vi "LSMcontroller_v66_improvedwfhandling.vi"() -> ()   [LabVIEW 2015] (continued)
                              }
                            }
                            n2122 = property on="Start" class="Bool (strict)"("Val(Sgnl)"=w5239) -> ()  [unwired: 2 in, 2 out]
                            n2123 = property on="Start" class="Bool (strict)"("Visible"=TRUE, "DisabledEnum"=T7."Enabled" ("Disabled")) -> ()  [unwired: 2 in, 2 out]
                            n2124 = property on="Stop" class="Bool (strict)"("Val(Sgnl)"=w5239) -> ()  [unwired: 2 in, 2 out]
                            n2125 = property on="Stop" class="Bool (strict)"("Visible"=FALSE, "DisabledEnum"=T7."Disabled" ("Disabled")) -> ()  [unwired: 2 in, 2 out]
                          }
                        }
                      }
                      frame Enabled {
                      }
                    }
                    n2126 = local write "64bit disabled"(TRUE ("64bit disabled")) -> ()
                  }
                }
              }
            }
          }
          event "avpp", "Angle ref", "xpixels ref", "Vx-min ref", "Vx-max ref", "ypixels ref", "Vy-min ref", "Vy-max ref", "ROI Type", "Sampling rate": Value Change {
            n2127 = event-data() -> ()  [unwired: 1 in, 6 out]
            n2128 = local read "avpp"() -> (w5258:i32)
            n2129 = local read "Angle ref"() -> (w5257:dbl)
            n2130 = local read "ROI Type"() -> (w5256:u16)
            n2131 = local read "xpixels ref"() -> (w5253:i32)
            n2132 = local read "Vx-min ref"() -> (w5252:dbl)
            n2133 = local read "Vx-max ref"() -> (w5251:dbl)
            n2134 = local read "ypixels ref"() -> (w5249:i32)
            n2135 = local read "Vy-min ref"() -> (w5250:dbl)
            n2136 = local read "Vy-max ref"() -> (w5246:dbl)
            n2137 = local read "Sampling rate"() -> (w5241:dbl)
            n2138 = local read "# of frames"() -> (w5245:i32)
            n2139 = local read "maxbufferAI"() -> (w5244:i32)
            n2140 = local read "Override AI buffer"() -> (w5242:bool)
            n2141 = call "2pparameters.vi"("command"="get") -> ("params out"=w5255:T10)  [unwired: 1 in]
            n2142 = Bundle By Name(cluster=w5255, "avpp"=w5258, "Angle Img"=w5257, "Xpixels Img"=w5253, "Vx-min Img"=w5252, "VX-max Img"=w5251, "Ypixels Img"=w5249, "Vy-min Img"=w5250, "Vy-max Img"=w5246, "srate"=w5241, "srate Img"=w5241, "measpoints"=w5245, "maxbufferAI"=w5244, "Drawing Mode"=w5256, "Vz-reset"=0.0, "AIoverride"=w5242) -> (w5247:T10)
            n2143 = call "2pparameters.vi"("Params in"=w5247, "command"="set") -> ()  [unwired: 1 out]
          }
          event "# of frames": Value Change {
            n2144 = event-data() -> ()  [unwired: 1 in, 6 out]
            n2145 = local read "Meastab"() -> (w5259:enum32{"X-Y Image", "Linescan", "Timetrace"})
            n2146 = case shown="\"X-Y Image\", Default" w5259 {
              frame "X-Y Image", Default {
                n2147 = local read "# of frames"() -> (w5260:i32)
                n2148 = call "2pparameters.vi"("command"="get") -> ("params out"=w5264:T10)  [unwired: 1 in]
                n2149 = Bundle By Name(cluster=w5264, "measpoints"=w5260) -> (w5261:T10)
                n2150 = call "2pparameters.vi"("Params in"=w5261, "command"="set") -> ()  [unwired: 1 out]
              }
              frame "Linescan" {
                n2151 = local read "srateAODOtt"() -> (w5274:dbl)
                n2152 = local read "# of frames"() -> (w5270:i32)
                n2153 = local read "refreshtime"() -> (w5276:dbl)
                n2154 = local read "bin"() -> (w5271:dbl)
                n2155 = call "tt_timeandsamples.vi"("bin"=w5271, "refreshtime"=w5276, "srateAODOtt"=w5274, "tot#ofsamples"=w5270) -> ("refreshrate"=w5273:dbl, "refreshbuffer"=w5272:i32, "timetracecycles"=w5269:i32)  [unwired: 5 in]
                n2156 = call "2pparameters.vi"("command"="get") -> ("params out"=w5266:T10)  [unwired: 1 in]
                n2157 = Bundle By Name(cluster=w5266, "measpoints"=w5270, "tt_cycles"=w5269, "refreshbuffer"=w5272, "refreshrate"=w5273) -> (w5268:T10)
                n2158 = Reciprocal(x=w5273) -> (1/x=w5275:dbl)
                n2159 = local write "refreshtime"(w5275) -> ()
                n2160 = call "2pparameters.vi"("Params in"=w5268, "command"="set") -> ()  [unwired: 1 out]
              }
              frame "Timetrace" {
                n2161 = local read "srateAODOtt"() -> (w5286:dbl)
                n2162 = local read "# of frames"() -> (w5282:i32)
                n2163 = local read "refreshtime"() -> (w5288:dbl)
                n2164 = local read "bin"() -> (w5283:dbl)
                n2165 = call "tt_timeandsamples.vi"("bin"=w5283, "refreshtime"=w5288, "srateAODOtt"=w5286, "tot#ofsamples"=w5282) -> ("refreshrate"=w5285:dbl, "refreshbuffer"=w5284:i32, "timetracecycles"=w5281:i32)  [unwired: 5 in]
                n2166 = call "2pparameters.vi"("command"="get") -> ("params out"=w5278:T10)  [unwired: 1 in]
                n2167 = Bundle By Name(cluster=w5278, "measpoints"=w5282, "tt_cycles"=w5281, "refreshbuffer"=w5284, "refreshrate"=w5285) -> (w5280:T10)
                n2168 = Reciprocal(x=w5285) -> (1/x=w5287:dbl)
                n2169 = local write "refreshtime"(w5287) -> ()
                n2170 = call "2pparameters.vi"("Params in"=w5280, "command"="set") -> ()  [unwired: 1 out]
              }
            }
          }
          event "srateAODOtt", "refreshtime", "Vx-ref", "Vy-ref", "Vx-min draw", "Vx-max draw", "Vy-min draw", "Vy-max draw", "bin": Value Change {
            n2171 = event-data() -> ()  [unwired: 1 in, 6 out]
            n2172 = local read "ypixels ref"() -> (w5320:i32)
            n2173 = local read "Vy-min draw"() -> (w5296:dbl)
            n2174 = local read "Vy-max draw"() -> (w5295:dbl)
            n2175 = local read "Vx-min draw"() -> (w5298:dbl)
            n2176 = local read "Vx-max draw"() -> (w5297:dbl)
            n2177 = local read "xpixels ref"() -> (w5294:i32)
            n2178 = local read "ROI Type"() -> (w5293:u16)
            n2179 = local read "Pel"() -> (w5292:dbl)
            n2180 = local read "srateAODOtt"() -> (w5302:dbl)
            n2181 = local read "# of frames"() -> (w5307:i32)
            n2182 = local read "refreshtime"() -> (w5300:dbl)
            n2183 = local read "bin"() -> (w5305:dbl)
            n2184 = local read "Override AI buffer"() -> (w5290:bool)
            n2185 = local read "finite samples"() -> (w5314:bool)
            n2186 = local read "srateAODOtt"() -> (w5289:dbl)
            n2187 = local read "srateAODOtt"() -> (w5308:dbl)
            n2188 = local read "continuous"() -> (w5313:bool)
            n2189 = local read "Angle ref"() -> (w5299:dbl)
            n2190 = local read "wavdet"() -> (w5315:bool)
            n2191 = local read "Vx-ref"() -> (w5310:dbl)
            n2192 = local read "Vy-ref"() -> (w5312:dbl)
            n2193 = local read "avpp"() -> (w5311:i32)
            n2194 = call "tt_timeandsamples.vi"("bin"=w5305, "refreshtime"=w5300, "srateAODOtt"=w5302, "tot#ofsamples"=w5307) -> ("refreshrate"=w5303:dbl, "refreshbuffer"=w5304:i32, "timetracecycles"=w5309:i32)  [unwired: 5 in]
            n2195 = local read "bin"() -> (w5306:dbl)
            n2196 = call "2pparameters.vi"("command"="get") -> ("params out"=w5318:T10)  [unwired: 1 in]
            n2197 = Bundle By Name(cluster=w5318, "Drawing Mode"=w5293, "measpoints"=w5307, "tt_cycles"=w5309, "refreshbuffer"=w5304, "refreshrate"=w5303, "Vx-ref"=w5310, "Vy-ref"=w5312, "srate"=w5289, "finite"=w5314, "cont"=w5313, "wavdet"=w5315, "avpp"=w5311, "srateAODO"=w5308, "bufferAI"=w5304, "bin"=w5306, "Angle Img"=w5299, "Vxminref"=w5298, "Vxmaxref"=w5297, "Vyminref"=w5296, "Vymaxref"=w5295, "Xpixels Img"=w5294, "Ypixels Img"=w5320, "Pel"=w5292, "Vz-reset"=0.0, "AIoverride"=w5290) -> (w5316:T10)
            n2198 = Reciprocal(x=w5303) -> (1/x=w5301:dbl)
            n2199 = local write "refreshtime"(w5301) -> ()
            n2200 = call "2pparameters.vi"("Params in"=w5316, "command"="set") -> ()  [unwired: 1 out]
          }
          event "Init": Value Change {
            # "Disabled for conversion to 64 bit"
            n2201 = event-data() -> ()  [unwired: 1 in, 6 out]
            n2202 = disable-structure shown="Disabled" {
              frame Disabled {
                n2203 = flat-sequence {
                  frame #0 {
                    n2204 = local read "Measurement"() -> (w5322:T4)
                    n2205 = case shown="\"Lifetime (scan)\", \"Lifetime (contour)\"" w5322 {
                      frame "X-Y-t movie", Default {
                      }
                      frame "Lifetime (point)" {
                        n2206 = stacked-sequence {
                          frame #0 {
                            n2207 = call "initialize.vi"("mode"=0) -> ()
                          }
                          frame #1 {
                            n2208 = call "calib.vi"() -> ()  [unwired: 1 in]
                          }
                        }
                      }
                      frame "Lifetime (scan)", "Lifetime (contour)" {
                        n2209 = stacked-sequence {
                          frame #0 {
                            n2210 = call "initialize.vi"("mode"=3) -> ()
                          }
                          frame #1 {
                            n2211 = call "calib.vi"() -> ()  [unwired: 1 in]
                          }
                        }
                      }
                    }
                  }
                  frame #1 {
                    n2212 = property on="Start" class="Bool (strict)"("Visible"=TRUE, "DisabledEnum"=T7."Enabled" ("Disabled")) -> ()  [unwired: 2 in, 2 out]
                    n2213 = property on="Init" class="Bool (strict)"("Visible"=FALSE, "DisabledEnum"=T7."Disabled and Grayed Out" ("Disabled"), "Value"=FALSE ("Init")) -> ()  [unwired: 2 in, 2 out]
                  }
                }
              }
              frame Enabled {
              }
            }
            n2214 = local write "64bit disabled"(TRUE ("64bit disabled")) -> ()
          }
          event "Measurement": Value Change {
            n2215 = event-data() -> ()  [unwired: 1 in, 5 out]
            n2216 = case shown="\"Lifetime (scan)\"" "Measurement" {
              frame "X-Y-t movie" {
                w5337 = T7."Disabled" ("Disabled")
                w5336 = FALSE ("Visible")
                n2217 = call "2pparameters.vi"("command"="get") -> ("params out"=w5347:T10)  [unwired: 1 in]
                n2218 = local write "graphtab"(T5."image" ("graphtab")) -> ()
                n2219 = local write "Save tab"(enum32{"withsave", "withoutsave"}."withsave" ("Save tab")) -> ()
                n2220 = Bundle By Name(cluster=w5347, "type"="X-Y-t movie") -> (w5345:T10)
                n2221 = call "2pparameters.vi"("Params in"=w5345, "command"="set") -> ()  [unwired: 1 out]
                n2222 = property on="refreshtime" class="DigNum (strict)"("Visible"=FALSE, "DisabledEnum"=T7."Disabled and Grayed Out" ("Disabled")) -> ()  [unwired: 2 in, 2 out]
                n2223 = property on="Start" class="Bool (strict)"("Visible"=TRUE, "DisabledEnum"=T7."Enabled" ("Disabled")) -> ()  [unwired: 2 in, 2 out]
                n2224 = property on="Init" class="Bool (strict)"("Visible"=FALSE, "DisabledEnum"=T7."Disabled and Grayed Out" ("Disabled"), "Value"=FALSE ("Init")) -> ()  [unwired: 2 in, 2 out]
                n2225 = property on="ttt" class="Enum (strict)"("Visible"=FALSE) -> ()  [unwired: 2 in, 2 out]
                n2226 = property on="# of frames" class="DigNum (strict)"("DisabledEnum"=T7."Enabled" ("Disabled"), "Caption.Text"="# of frames") -> ()  [unwired: 2 in, 2 out]
                n2227 = property on="continuous" class="Bool (strict)"("Visible"=TRUE, "DisabledEnum"=T7."Enabled" ("Disabled")) -> ()  [unwired: 2 in, 2 out]
                n2228 = property on="finite samples" class="Bool (strict)"("Visible"=TRUE, "DisabledEnum"=T7."Enabled" ("Disabled")) -> ()  [unwired: 2 in, 2 out]
                n2229 = property on="avpp" class="DigNum (strict)"("Visible"=TRUE, "DisabledEnum"=T7."Enabled" ("Disabled")) -> ()  [unwired: 2 in, 2 out]
                n2230 = property on="srateAODOtt" class="DigNum (strict)"("Visible"=FALSE, "DisabledEnum"=T7."Disabled" ("Disabled")) -> ()  [unwired: 2 in, 2 out]
                n2231 = local write "save\ndata"(TRUE ("save\ndata")) -> ()
                n2232 = property on="finite samples" class="Bool (strict)"("Val(Sgnl)"=TRUE ("continuous for display")) -> ()  [unwired: 2 in, 2 out]
                n2233 = property on="continuous" class="Bool (strict)"("Value"=FALSE ("continuous for display")) -> ()  [unwired: 2 in, 2 out]
                n2234 = property on="Current Average" class="DigNum (strict)"("Visible"=TRUE, "DisabledEnum"=T7."Enabled" ("Disabled")) -> ()  [unwired: 2 in, 2 out]
                n2235 = property on="img_CH1" class="IntGraph (strict)"("ZScale.Maximum"=7.0 ("Z Scale.Range:Maximum")) -> ()  [unwired: 2 in, 2 out]
                n2236 = property on="Sampling rate" class="DigNum (strict)"("Visible"=TRUE, "DisabledEnum"=T7."Enabled" ("Disabled")) -> ()  [unwired: 2 in, 2 out]
                n2237 = property on="Pel" class="DigNum (strict)"("Visible"=w5336, "DisabledEnum"=w5337) -> ()  [unwired: 2 in, 2 out]
                n2238 = property on="bin" class="DigNum (strict)"("Visible"=w5336, "DisabledEnum"=w5337) -> ()  [unwired: 2 in, 2 out]
                "Meastab" <- enum32{"X-Y Image", "Linescan", "Timetrace"}."X-Y Image" ("Meastab")
                "Zscantab" <- enum32{"withzscan", "withoutzscan", "lifetime"}."withoutzscan" ("Zscantab")
              }
              frame "X-Y-Z stack" {
                w5374 = T7."Disabled" ("Disabled")
                w5373 = FALSE ("Visible")
                n2239 = call "2pparameters.vi"("command"="get") -> ("params out"=w5384:T10)  [unwired: 1 in]
                n2240 = call "2pparameters.vi"("command"="get") -> ("params out"=w5388:T10)  [unwired: 1 in]
                n2241 = Bundle By Name(cluster=w5384, "type"="X-Y-Z stack") -> (w5382:T10)
                n2242 = Unbundle By Name(w5388) -> ("motorref"=w5387:refnum<k7>)
                n2243 = call "2pparameters.vi"("Params in"=w5382, "command"="set") -> ()  [unwired: 1 out]
                n2244 = local write "Zscantab"(enum32{"withzscan", "withoutzscan", "lifetime"}."withzscan" ("Zscantab")) -> ()
                n2245 = local write "Meastab"(enum32{"X-Y Image", "Linescan", "Timetrace"}."X-Y Image" ("Meastab")) -> ()
                n2246 = invoke class="MG17Motor" method="GetPosition"(reference=w5387, "lChanID"=0, "pfPosition"=sgl 0.0) -> ("pfPosition"=w5399:sgl)  [unwired: 2 in, 4 out]
                n2247 = property on="refreshtime" class="DigNum (strict)"("Visible"=FALSE, "DisabledEnum"=T7."Disabled and Grayed Out" ("Disabled")) -> ()  [unwired: 2 in, 2 out]
                n2248 = property on="Start" class="Bool (strict)"("Visible"=TRUE, "DisabledEnum"=T7."Enabled" ("Disabled")) -> ()  [unwired: 2 in, 2 out]
                n2249 = property on="Init" class="Bool (strict)"("Visible"=FALSE, "DisabledEnum"=T7."Disabled and Grayed Out" ("Disabled"), "Value"=FALSE ("Init")) -> ()  [unwired: 2 in, 2 out]
                n2250 = property on="ttt" class="Enum (strict)"("Visible"=FALSE) -> ()  [unwired: 2 in, 2 out]
                n2251 = Multiply(x=w5399, y=1000.0) -> (x*y=w5398:dbl)
                n2252 = local write "Actual Z position"(w5398) -> ()
                n2253 = local write "Save tab"(enum32{"withsave", "withoutsave"}."withsave" ("Save tab")) -> ()
                n2254 = property on="finite samples" class="Bool (strict)"("Visible"=FALSE, "DisabledEnum"=T7."Disabled and Grayed Out" ("Disabled")) -> ()  [unwired: 2 in, 2 out]
                n2255 = property on="avpp" class="DigNum (strict)"("Visible"=TRUE, "DisabledEnum"=T7."Enabled" ("Disabled")) -> ()  [unwired: 2 in, 2 out]
                n2256 = property on="continuous" class="Bool (strict)"("Visible"=FALSE, "DisabledEnum"=T7."Disabled and Grayed Out" ("Disabled")) -> ()  [unwired: 2 in, 2 out]
                n2257 = property on="img_CH1" class="IntGraph (strict)"("ZScale.Maximum"=7.0 ("Z Scale.Range:Maximum")) -> ()  [unwired: 2 in, 2 out]
                n2258 = property on="srateAODOtt" class="DigNum (strict)"("Visible"=FALSE, "DisabledEnum"=T7."Disabled" ("Disabled")) -> ()  [unwired: 2 in, 2 out]
                n2259 = property on="Pel" class="DigNum (strict)"("Visible"=w5373, "DisabledEnum"=w5374) -> ()  [unwired: 2 in, 2 out]
                n2260 = property on="bin" class="DigNum (strict)"("Visible"=w5373, "DisabledEnum"=w5374) -> ()  [unwired: 2 in, 2 out]
                n2261 = property on="Current Average" class="DigNum (strict)"("Visible"=TRUE, "DisabledEnum"=T7."Enabled" ("Disabled")) -> ()  [unwired: 2 in, 2 out]
                n2262 = property on="# of frames" class="DigNum (strict)"("Caption.Text"="# of slices", "DisabledEnum"=T7."Disabled and Grayed Out" ("Disabled")) -> ()  [unwired: 2 in, 2 out]
                n2263 = local write "save\ndata"(TRUE ("save\ndata")) -> ()
                n2264 = property on="finite samples" class="Bool (strict)"("Val(Sgnl)"=TRUE ("continuous for display")) -> ()  [unwired: 2 in, 2 out]
                n2265 = property on="continuous" class="Bool (strict)"("Value"=FALSE ("continuous for display")) -> ()  [unwired: 2 in, 2 out]
                n2266 = property on="Sampling rate" class="DigNum (strict)"("Visible"=TRUE, "DisabledEnum"=T7."Enabled" ("Disabled")) -> ()  [unwired: 2 in, 2 out]
              }
              frame "X-Y-Z-t movie" {
                w5418 = T7."Disabled" ("Disabled")
                w5417 = FALSE ("Visible")
                n2267 = property on="# of frames" class="DigNum (strict)"("DisabledEnum"=T7."Enabled" ("Disabled")) -> ()  [unwired: 2 in, 2 out]
                n2268 = property on="Current Average" class="DigNum (strict)"("Visible"=TRUE, "DisabledEnum"=T7."Enabled" ("Disabled")) -> ()  [unwired: 2 in, 2 out]
                n2269 = property on="avpp" class="DigNum (strict)"("Visible"=TRUE, "DisabledEnum"=T7."Enabled" ("Disabled")) -> ()  [unwired: 2 in, 2 out]
                n2270 = local write "Save tab"(enum32{"withsave", "withoutsave"}."withsave" ("Save tab")) -> ()
                n2271 = local write "Zscantab"(enum32{"withzscan", "withoutzscan", "lifetime"}."withzscan" ("Zscantab")) -> ()
                n2272 = local write "Meastab"(enum32{"X-Y Image", "Linescan", "Timetrace"}."X-Y Image" ("Meastab")) -> ()
                n2273 = property on="Start" class="Bool (strict)"("Visible"=TRUE, "DisabledEnum"=T7."Enabled" ("Disabled")) -> ()  [unwired: 2 in, 2 out]
                n2274 = property on="refreshtime" class="DigNum (strict)"("Visible"=FALSE, "DisabledEnum"=T7."Disabled and Grayed Out" ("Disabled")) -> ()  [unwired: 2 in, 2 out]
                n2275 = property on="Init" class="Bool (strict)"("Visible"=FALSE, "DisabledEnum"=T7."Disabled and Grayed Out" ("Disabled"), "Value"=FALSE ("Init")) -> ()  [unwired: 2 in, 2 out]
                n2276 = property on="ttt" class="Enum (strict)"("Visible"=FALSE) -> ()  [unwired: 2 in, 2 out]
                n2277 = call "2pparameters.vi"("command"="get") -> ("params out"=w5428:T10)  [unwired: 1 in]
                n2278 = Bundle By Name(cluster=w5428, "type"="X-Y-Z-t movie") -> (w5426:T10)
                n2279 = property on="continuous" class="Bool (strict)"("Visible"=TRUE, "DisabledEnum"=T7."Enabled" ("Disabled")) -> ()  [unwired: 2 in, 2 out]
                n2280 = property on="finite samples" class="Bool (strict)"("Visible"=TRUE, "DisabledEnum"=T7."Enabled" ("Disabled")) -> ()  [unwired: 2 in, 2 out]
                n2281 = call "2pparameters.vi"("Params in"=w5426, "command"="set") -> ()  [unwired: 1 out]
                n2282 = property on="srateAODOtt" class="DigNum (strict)"("Visible"=FALSE, "DisabledEnum"=T7."Disabled" ("Disabled")) -> ()  [unwired: 2 in, 2 out]
                n2283 = local write "save\ndata"(TRUE ("save\ndata")) -> ()
                n2284 = property on="img_CH1" class="IntGraph (strict)"("ZScale.Maximum"=7.0 ("Z Scale.Range:Maximum")) -> ()  [unwired: 2 in, 2 out]
                n2285 = property on="continuous" class="Bool (strict)"("Value"=FALSE ("continuous for display")) -> ()  [unwired: 2 in, 2 out]
                n2286 = property on="finite samples" class="Bool (strict)"("Value"=TRUE ("continuous for display")) -> ()  [unwired: 2 in, 2 out]
                n2287 = property on="Sampling rate" class="DigNum (strict)"("Visible"=TRUE, "DisabledEnum"=T7."Enabled" ("Disabled")) -> ()  [unwired: 2 in, 2 out]
                n2288 = property on="Pel" class="DigNum (strict)"("Visible"=w5417, "DisabledEnum"=w5418) -> ()  [unwired: 2 in, 2 out]
                n2289 = property on="bin" class="DigNum (strict)"("Visible"=w5417, "DisabledEnum"=w5418) -> ()  [unwired: 2 in, 2 out]
              }
              frame "linescan" {
                w5453 = T7."Enabled" ("Disabled")
                w5452 = TRUE ("Visible")
                w5455 = T7."Enabled" ("Disabled")
                w5454 = TRUE ("Visible")
                n2290 = local write "Meastab"(enum32{"X-Y Image", "Linescan", "Timetrace"}."Linescan" ("Meastab")) -> ()
                n2291 = property on="Current Average" class="DigNum (strict)"("Visible"=TRUE, "DisabledEnum"=T7."Enabled" ("Disabled")) -> ()  [unwired: 2 in, 2 out]
                n2292 = property on="ttt" class="Enum (strict)"("Visible"=FALSE) -> ()  [unwired: 2 in, 2 out]
                n2293 = local write "Save tab"(enum32{"withsave", "withoutsave"}."withsave" ("Save tab")) -> ()
                n2294 = local write "Zscantab"(enum32{"withzscan", "withoutzscan", "lifetime"}."withoutzscan" ("Zscantab")) -> ()
                n2295 = property on="refreshtime" class="DigNum (strict)"("Visible"=FALSE, "DisabledEnum"=T7."Disabled and Grayed Out" ("Disabled")) -> ()  [unwired: 2 in, 2 out]
                n2296 = property on="continuous" class="Bool (strict)"("Value"=FALSE ("continuous for display")) -> ()  [unwired: 2 in, 2 out]
                n2297 = property on="finite samples" class="Bool (strict)"("Value"=TRUE ("continuous for display")) -> ()  [unwired: 2 in, 2 out]
                n2298 = local write "save\ndata"(TRUE ("save\ndata")) -> ()
                n2299 = property on="Start" class="Bool (strict)"("Visible"=TRUE, "DisabledEnum"=T7."Enabled" ("Disabled")) -> ()  [unwired: 2 in, 2 out]
                n2300 = property on="Init" class="Bool (strict)"("Visible"=FALSE, "DisabledEnum"=T7."Disabled and Grayed Out" ("Disabled"), "Value"=FALSE ("Init")) -> ()  [unwired: 2 in, 2 out]
                n2301 = call "2pparameters.vi"("command"="get") -> ("params out"=w5464:T10)  [unwired: 1 in]
                n2302 = Bundle By Name(cluster=w5464, "type"="linescan") -> (w5462:T10)
                n2303 = property on="# of frames" class="DigNum (strict)"("DisabledEnum"=T7."Enabled" ("Disabled"), "Caption.Text"="# of lines") -> ()  [unwired: 2 in, 2 out]
                n2304 = property on="continuous" class="Bool (strict)"("Visible"=TRUE, "DisabledEnum"=T7."Enabled" ("Disabled")) -> ()  [unwired: 2 in, 2 out]
                n2305 = property on="avpp" class="DigNum (strict)"("Visible"=TRUE, "DisabledEnum"=T7."Enabled" ("Disabled")) -> ()  [unwired: 2 in, 2 out]
                n2306 = property on="finite samples" class="Bool (strict)"("Visible"=TRUE, "DisabledEnum"=T7."Enabled" ("Disabled")) -> ()  [unwired: 2 in, 2 out]
                n2307 = property on="srateAODOtt" class="DigNum (strict)"("Visible"=TRUE, "DisabledEnum"=T7."Enabled" ("Disabled")) -> ()  [unwired: 2 in, 2 out]
                n2308 = call "2pparameters.vi"("Params in"=w5462, "command"="set") -> ()  [unwired: 1 out]
                n2309 = property on="Pel" class="DigNum (strict)"("Visible"=w5454, "DisabledEnum"=w5455) -> ()  [unwired: 2 in, 2 out]
                n2310 = property on="bin" class="DigNum (strict)"("Visible"=w5454, "DisabledEnum"=w5455) -> ()  [unwired: 2 in, 2 out]
                n2311 = property on="Sampling rate" class="DigNum (strict)"("Visible"=FALSE, "DisabledEnum"=T7."Disabled" ("Disabled")) -> ()  [unwired: 2 in, 2 out]
                n2312 = property on="Pel" class="DigNum (strict)"("Visible"=w5452, "DisabledEnum"=w5453) -> ()  [unwired: 2 in, 2 out]
                n2313 = property on="bin" class="DigNum (strict)"("Visible"=w5452, "DisabledEnum"=w5453) -> ()  [unwired: 2 in, 2 out]
              }
              frame "Timetrace" {
                w5490 = T7."Enabled" ("Disabled")
                w5489 = TRUE ("Visible")
                n2314 = call "2pparameters.vi"("command"="get") -> ("params out"=w5495:T10)  [unwired: 1 in]
                n2315 = local write "Meastab"(enum32{"X-Y Image", "Linescan", "Timetrace"}."Timetrace" ("Meastab")) -> ()
                n2316 = Unbundle By Name(w5495) -> ("Angle draw"=w5497:dbl)
                n2317 = local write "Zscantab"(enum32{"withzscan", "withoutzscan", "lifetime"}."withoutzscan" ("Zscantab")) -> ()
                n2318 = property on="# of frames" class="DigNum (strict)"("DisabledEnum"=T7."Enabled" ("Disabled"), "Caption.Text"="# of samples") -> ()  [unwired: 2 in, 2 out]
                n2319 = property on="refreshtime" class="DigNum (strict)"("Visible"=TRUE, "DisabledEnum"=T7."Enabled" ("Disabled")) -> ()  [unwired: 2 in, 2 out]
                n2320 = property on="avpp" class="DigNum (strict)"("Visible"=FALSE, "DisabledEnum"=T7."Disabled and Grayed Out" ("Disabled")) -> ()  [unwired: 2 in, 2 out]
                n2321 = property on="Current Average" class="DigNum (strict)"("Visible"=FALSE, "DisabledEnum"=T7."Disabled and Grayed Out" ("Disabled")) -> ()  [unwired: 2 in, 2 out]
                n2322 = local write "Angle drawing"(w5497) -> ()
                n2323 = property on="ttt" class="Enum (strict)"("Visible"=TRUE) -> ()  [unwired: 2 in, 2 out]
                n2324 = property on="continuous" class="Bool (strict)"("Visible"=TRUE, "DisabledEnum"=T7."Enabled" ("Disabled")) -> ()  [unwired: 2 in, 2 out]
                n2325 = property on="finite samples" class="Bool (strict)"("Visible"=TRUE, "DisabledEnum"=T7."Enabled" ("Disabled")) -> ()  [unwired: 2 in, 2 out]
                n2326 = local write "save\ndata"(TRUE ("save\ndata")) -> ()
                n2327 = property on="finite samples" class="Bool (strict)"("Val(Sgnl)"=TRUE ("continuous for display")) -> ()  [unwired: 2 in, 2 out]
                n2328 = property on="continuous" class="Bool (strict)"("Value"=FALSE ("continuous for display")) -> ()  [unwired: 2 in, 2 out]
                n2329 = local write "Save tab"(enum32{"withsave", "withoutsave"}."withsave" ("Save tab")) -> ()
                n2330 = property on="srateAODOtt" class="DigNum (strict)"("Visible"=TRUE, "DisabledEnum"=T7."Enabled" ("Disabled")) -> ()  [unwired: 2 in, 2 out]
                n2331 = call "2pparameters.vi"("command"="get") -> ("params out"=w5502:T10)  [unwired: 1 in]
                n2332 = property on="Start" class="Bool (strict)"("Visible"=TRUE, "DisabledEnum"=T7."Enabled" ("Disabled")) -> ()  [unwired: 2 in, 2 out]
                n2333 = property on="Init" class="Bool (strict)"("Visible"=FALSE, "DisabledEnum"=T7."Disabled and Grayed Out" ("Disabled"), "Value"=FALSE ("Init")) -> ()  [unwired: 2 in, 2 out]
                n2334 = Bundle By Name(cluster=w5502, "type"="Timetrace") -> (w5500:T10)
                n2335 = property on="Sampling rate" class="DigNum (strict)"("Visible"=FALSE, "DisabledEnum"=T7."Disabled" ("Disabled")) -> ()  [unwired: 2 in, 2 out]
                n2336 = property on="Pel" class="DigNum (strict)"("Visible"=w5489, "DisabledEnum"=w5490) -> ()  [unwired: 2 in, 2 out]
                n2337 = property on="bin" class="DigNum (strict)"("Visible"=w5489, "DisabledEnum"=w5490) -> ()  [unwired: 2 in, 2 out]
                n2338 = call "2pparameters.vi"("Params in"=w5500, "command"="set") -> ()  [unwired: 1 out]
              }
              frame "Lifetime (point)" {
                w5523 = T7."Enabled" ("Disabled")
                w5522 = TRUE ("Visible")
                n2339 = property on="Pel" class="DigNum (strict)"("Visible"=w5522, "DisabledEnum"=w5523) -> ()  [unwired: 2 in, 2 out]
                n2340 = property on="bin" class="DigNum (strict)"("Visible"=w5522, "DisabledEnum"=w5523) -> ()  [unwired: 2 in, 2 out]
                n2341 = property on="ttt" class="Enum (strict)"("Visible"=FALSE) -> ()  [unwired: 2 in, 2 out]
                n2342 = local write "Zscantab"(enum32{"withzscan", "withoutzscan", "lifetime"}."lifetime" ("Zscantab")) -> ()
                n2343 = local write "graphtab"(T5."Lifetime" ("graphtab")) -> ()
                n2344 = local write "Meastab"(enum32{"X-Y Image", "Linescan", "Timetrace"}."Timetrace" ("Meastab")) -> ()
                n2345 = call "lifetimeparameters.vi"("command"="get") -> ("Params out"=w5530:T19)  [unwired: 1 in]
                n2346 = Unbundle By Name(w5530) -> ("initialized"=w5531:bool)
                n2347 = property on="srateAODOtt" class="DigNum (strict)"("Visible"=TRUE, "DisabledEnum"=T7."Enabled" ("Disabled")) -> ()  [unwired: 2 in, 2 out]
                n2348 = case shown="False" w5531 {
                  frame False {
                    n2349 = property on="Init" class="Bool (strict)"("Visible"=TRUE, "DisabledEnum"=T7."Enabled" ("Disabled")) -> ()  [unwired: 2 in, 2 out]
                    n2350 = property on="Start" class="Bool (strict)"("Visible"=FALSE, "DisabledEnum"=T7."Disabled and Grayed Out" ("Disabled")) -> ()  [unwired: 2 in, 2 out]
                  }
                  frame True {
                  }
                }
                n2351 = property on="Sampling rate" class="DigNum (strict)"("Visible"=FALSE, "DisabledEnum"=T7."Disabled" ("Disabled")) -> ()  [unwired: 2 in, 2 out]
              }
              frame "Lifetime (scan)" {
                w5540 = T7."Disabled" ("Disabled")
                w5539 = FALSE ("Visible")
                n2352 = call "lifetimeparameters.vi"("command"="get") -> ("Params out"=w5552:T19)  [unwired: 1 in]
                n2353 = local write "graphtab"(T5."image" ("graphtab")) -> ()
                n2354 = local write "Save tab"(enum32{"withsave", "withoutsave"}."withsave" ("Save tab")) -> ()
                n2355 = local write "Meastab"(enum32{"X-Y Image", "Linescan", "Timetrace"}."X-Y Image" ("Meastab")) -> ()
                n2356 = local write "Zscantab"(enum32{"withzscan", "withoutzscan", "lifetime"}."lifetime" ("Zscantab")) -> ()
                n2357 = Unbundle By Name(w5552) -> ("initialized"=w5551:bool)
                n2358 = property on="ttt" class="Enum (strict)"("Visible"=FALSE) -> ()  [unwired: 2 in, 2 out]
                n2359 = property on="refreshtime" class="DigNum (strict)"("Visible"=FALSE, "DisabledEnum"=T7."Disabled and Grayed Out" ("Disabled")) -> ()  [unwired: 2 in, 2 out]
                n2360 = property on="Pel" class="DigNum (strict)"("Visible"=w5539, "DisabledEnum"=w5540) -> ()  [unwired: 2 in, 2 out]
                n2361 = property on="bin" class="DigNum (strict)"("Visible"=w5539, "DisabledEnum"=w5540) -> ()  [unwired: 2 in, 2 out]
                n2362 = property on="save data" class="Bool (strict)"("Visible"=TRUE, "DisabledEnum"=T7."Enabled" ("Disabled"), "Value"=TRUE ("Visible")) -> ()  [unwired: 2 in, 2 out]
                n2363 = case shown="False" w5551 {
                  frame False {
                    n2364 = property on="Init" class="Bool (strict)"("Visible"=TRUE, "DisabledEnum"=T7."Enabled" ("Disabled")) -> ()  [unwired: 2 in, 2 out]
                    n2365 = property on="Start" class="Bool (strict)"("Visible"=FALSE, "DisabledEnum"=T7."Disabled and Grayed Out" ("Disabled")) -> ()  [unwired: 2 in, 2 out]
                  }
                  frame True {
                  }
                }
                n2366 = call "2pparameters.vi"("command"="get") -> ("params out"=w5557:T10)  [unwired: 1 in]
                n2367 = property on="continuous" class="Bool (strict)"("Visible"=TRUE, "DisabledEnum"=T7."Disabled and Grayed Out" ("Disabled")) -> ()  [unwired: 2 in, 2 out]
                n2368 = property on="finite samples" class="Bool (strict)"("Visible"=TRUE, "DisabledEnum"=T7."Enabled" ("Disabled")) -> ()  [unwired: 2 in, 2 out]
                n2369 = Bundle By Name(cluster=w5557, "type"="Lifetime (scan)") -> (w5555:T10)
                n2370 = call "2pparameters.vi"("Params in"=w5555, "command"="set") -> ()  [unwired: 1 out]
                n2371 = property on="finite samples" class="Bool (strict)"("Val(Sgnl)"=TRUE ("continuous for display")) -> ()  [unwired: 2 in, 2 out]
                n2372 = property on="continuous" class="Bool (strict)"("Value"=FALSE ("continuous for display")) -> ()  [unwired: 2 in, 2 out]
                n2373 = property on="srateAODOtt" class="DigNum (strict)"("Visible"=FALSE, "DisabledEnum"=T7."Disabled" ("Disabled")) -> ()  [unwired: 2 in, 2 out]
                n2374 = property on="# of frames" class="DigNum (strict)"("DisabledEnum"=T7."Enabled" ("Disabled"), "Caption.Text"="# of frames") -> ()  [unwired: 2 in, 2 out]
                n2375 = property on="img_CH1" class="IntGraph (strict)"("ZScale.Maximum"=12.5 ("Z Scale.Range:Maximum")) -> ()  [unwired: 2 in, 2 out]
                n2376 = property on="Current Average" class="DigNum (strict)"("Visible"=TRUE, "DisabledEnum"=T7."Enabled" ("Disabled")) -> ()  [unwired: 2 in, 2 out]
                n2377 = property on="Sampling rate" class="DigNum (strict)"("Visible"=TRUE, "DisabledEnum"=T7."Enabled" ("Disabled")) -> ()  [unwired: 2 in, 2 out]
                n2378 = property on="avpp" class="DigNum (strict)"("Visible"=TRUE, "DisabledEnum"=T7."Enabled" ("Disabled")) -> ()  [unwired: 2 in, 2 out]
              }
              frame "Lifetime (contour)" {
                w5581 = T7."Enabled" ("Disabled")
                w5580 = TRUE ("Visible")
                n2379 = call "2pparameters.vi"("command"="get") -> ("params out"=w5588:T10)  [unwired: 1 in]
                n2380 = property on="# of frames" class="DigNum (strict)"("DisabledEnum"=T7."Enabled" ("Disabled"), "Caption.Text"="# of samples") -> ()  [unwired: 2 in, 2 out]
                n2381 = property on="refreshtime" class="DigNum (strict)"("Visible"=TRUE, "DisabledEnum"=T7."Enabled" ("Disabled")) -> ()  [unwired: 2 in, 2 out]
                n2382 = Unbundle By Name(w5588) -> ("Angle draw"=w5590:dbl)
                n2383 = property on="avpp" class="DigNum (strict)"("Visible"=FALSE, "DisabledEnum"=T7."Disabled and Grayed Out" ("Disabled")) -> ()  [unwired: 2 in, 2 out]
                n2384 = property on="Current Average" class="DigNum (strict)"("Visible"=FALSE, "DisabledEnum"=T7."Disabled and Grayed Out" ("Disabled")) -> ()  [unwired: 2 in, 2 out]
                n2385 = local write "Angle drawing"(w5590) -> ()
                n2386 = local write "Save tab"(enum32{"withsave", "withoutsave"}."withsave" ("Save tab")) -> ()
                n2387 = local write "Zscantab"(enum32{"withzscan", "withoutzscan", "lifetime"}."lifetime" ("Zscantab")) -> ()
                n2388 = local write "graphtab"(T5."Lifetime" ("graphtab")) -> ()
                n2389 = local write "Meastab"(enum32{"X-Y Image", "Linescan", "Timetrace"}."Timetrace" ("Meastab")) -> ()
                n2390 = property on="ttt" class="Enum (strict)"("Visible"=TRUE) -> ()  [unwired: 2 in, 2 out]
                n2391 = call "lifetimeparameters.vi"("command"="get") -> ("Params out"=w5612:T19)  [unwired: 1 in]
                n2392 = property on="finite samples" class="Bool (strict)"("Val(Sgnl)"=TRUE ("continuous for display")) -> ()  [unwired: 2 in, 2 out]
                n2393 = local write "save\ndata"(TRUE ("save\ndata")) -> ()
                n2394 = Unbundle By Name(w5612) -> ("initialized"=w5613:bool)
                n2395 = property on="continuous" class="Bool (strict)"("Visible"=TRUE, "DisabledEnum"=T7."Enabled" ("Disabled")) -> ()  [unwired: 2 in, 2 out]
                n2396 = property on="finite samples" class="Bool (strict)"("Visible"=TRUE, "DisabledEnum"=T7."Enabled" ("Disabled")) -> ()  [unwired: 2 in, 2 out]
                n2397 = property on="Pel" class="DigNum (strict)"("Visible"=w5580, "DisabledEnum"=w5581) -> ()  [unwired: 2 in, 2 out]
                n2398 = property on="bin" class="DigNum (strict)"("Visible"=w5580, "DisabledEnum"=w5581) -> ()  [unwired: 2 in, 2 out]
                n2399 = property on="continuous" class="Bool (strict)"("Value"=FALSE ("continuous for display")) -> ()  [unwired: 2 in, 2 out]
                n2400 = case shown="False" w5613 {
                  frame False {
                    n2401 = property on="Init" class="Bool (strict)"("Visible"=TRUE, "DisabledEnum"=T7."Enabled" ("Disabled")) -> ()  [unwired: 2 in, 2 out]
                    n2402 = property on="Start" class="Bool (strict)"("Visible"=FALSE, "DisabledEnum"=T7."Disabled and Grayed Out" ("Disabled")) -> ()  [unwired: 2 in, 2 out]
                  }
                  frame True {
                  }
                }
                n2403 = property on="srateAODOtt" class="DigNum (strict)"("Visible"=TRUE, "DisabledEnum"=T7."Enabled" ("Disabled")) -> ()  [unwired: 2 in, 2 out]
                n2404 = call "2pparameters.vi"("command"="get") -> ("params out"=w5592:T10)  [unwired: 1 in]
                n2405 = Bundle By Name(cluster=w5592, "type"="Timetrace") -> (w5586:T10)
                n2406 = call "2pparameters.vi"("Params in"=w5586, "command"="set") -> ()  [unwired: 1 out]
                n2407 = property on="Sampling rate" class="DigNum (strict)"("Visible"=FALSE, "DisabledEnum"=T7."Disabled" ("Disabled")) -> ()  [unwired: 2 in, 2 out]
              }
            }
          }
          event "Laserpower \n(%)": Value Change {
            n2408 = event-data() -> ("OldVal"=w5621:dbl, "NewVal"=w5622:dbl)  [unwired: 1 in, 4 out]
            n2409 = Not Equal?(x=w5621, y=w5622) -> (x != y?=w5623:bool)
            n2410 = case shown="True" w5623 {
              tunnel: w5622 -> [_ w5625]
              frame False {
              }
              frame True {
                n2411 = local read "wavelength(nm)"() -> (w5626:dbl)
                n2412 = call "configuration.vi"("command"="get") -> ("config out"=w5630:T11)  [unwired: 2 in, 1 out]
                n2413 = call "pockelscellcalibration.vi"("l"=w5626, "T"=w5625) -> ("Vout"=w5624:dbl)
                n2414 = Unbundle By Name(w5630) -> ("Vto2P"=w5629:i32, "AOlines"=w5628:tag[])
                n2415 = property on="lpow" class="DigNum (strict)"("Value"=w5625) -> ()  [unwired: 2 in, 2 out]
                n2416 = local write "Vpockels"(w5624) -> ()
                n2417 = Index Array(array=w5628, index=w5629) -> (element=w5627:tag)
                n2418 = call-poly <vilib>:"DAQmx Create Virtual Channel.vi"("physical channels"=w5627) -> ("task out"=w5633:refnum<k21>, "error out"=w5632:errorcluster)  [unwired: 13 in]
                n2419 = call-poly <vilib>:"DAQmx Write.vi"("task/channels in"=w5633, "data"=w5624, "error in"=w5632) -> ("task out"=w5634:refnum<k21>, "error out"=w5635:errorcluster)  [unwired: 10 in, 1 out]
                n2420 = call <vilib>:"DAQmx Start Task.vi"("task/channels in"=w5634, "error in"=w5635) -> ("task out"=w5636:refnum<k21>, "error out"=w5637:errorcluster)  [unwired: 12 in]
                n2421 = call <vilib>:"DAQmx Stop Task.vi"("task/channels in"=w5636, "error in"=w5637) -> ("task out"=w5638:refnum<k21>, "error out"=w5639:errorcluster)  [unwired: 12 in]
                n2422 = call <vilib>:"DAQmx Clear Task.vi"("task in"=w5638, "error in"=w5639) -> ()  [unwired: 13 in, 1 out]
              }
            }
          }
          event "lpow": Value Change {
            n2423 = event-data() -> ("OldVal"=w5640:dbl, "NewVal"=w5641:dbl)  [unwired: 1 in, 4 out]
            n2424 = Not Equal?(x=w5640, y=w5641) -> (x != y?=w5642:bool)
            n2425 = case shown="True" w5642 {
              tunnel: w5641 -> [_ w5645]
              frame False {
              }
              frame True {
                n2426 = local read "wavelength(nm)"() -> (w5644:dbl)
                n2427 = call "pockelscellcalibration.vi"("l"=w5644, "T"=w5645) -> ("Vout"=w5643:dbl)
                n2428 = call "configuration.vi"("command"="get") -> ("config out"=w5649:T11)  [unwired: 2 in, 1 out]
                n2429 = Unbundle By Name(w5649) -> ("Vto2P"=w5648:i32, "AOlines"=w5647:tag[])
                n2430 = local write "Vpockels"(w5643) -> ()
                n2431 = property on="Laserpower \n(%)" class="Slide (strict)"("Value"=w5645) -> ()  [unwired: 2 in, 2 out]
                n2432 = Index Array(array=w5647, index=w5648) -> (element=w5646:tag)
                n2433 = call-poly <vilib>:"DAQmx Create Virtual Channel.vi"("physical channels"=w5646) -> ("task out"=w5652:refnum<k21>, "error out"=w5651:errorcluster)  [unwired: 13 in]
                n2434 = call-poly <vilib>:"DAQmx Write.vi"("task/channels in"=w5652, "data"=w5643, "error in"=w5651) -> ("task out"=w5653:refnum<k21>, "error out"=w5654:errorcluster)  [unwired: 10 in, 1 out]
                n2435 = call <vilib>:"DAQmx Start Task.vi"("task/channels in"=w5653, "error in"=w5654) -> ("task out"=w5655:refnum<k21>, "error out"=w5656:errorcluster)  [unwired: 12 in]
                n2436 = call <vilib>:"DAQmx Stop Task.vi"("task/channels in"=w5655, "error in"=w5656) -> ("task out"=w5657:refnum<k21>, "error out"=w5658:errorcluster)  [unwired: 12 in]
                n2437 = call <vilib>:"DAQmx Clear Task.vi"("task in"=w5657, "error in"=w5658) -> ()  [unwired: 13 in, 1 out]
              }
            }
          }
          event "sealtest": Value Change {
            n2438 = event-data() -> ()  [unwired: 1 in, 6 out]
            n2439 = case shown="True" "sealtest" {
              frame False {
              }
              frame True {
                n2440 = stacked-sequence {
                  seq-local: [w5660 _ _ _ _ _ _] -> [_ w5693 _ w5745 _ _ _]
                  frame #0 {
                    n2441 = stacked-sequence {
                      tunnel: [_ w5672 _] -> w5660
                      frame #0 {
                        n2442 = call "2pparameters.vi"("command"="get") -> ("params out"=w5665:T10)  [unwired: 1 in]
                        n2443 = Unbundle By Name(w5665) -> ("autoshutter"=w5666:bool)
                        n2444 = local read "OCchecked?"() -> (w5663:bool)
                        n2445 = call "sealtestwfparams.vi"("command"="set") -> ()  [unwired: 6 in, 1 out]
                        n2446 = case shown="False" w5663 {
                          frame False {
                            n2447 = One Button Dialog(message="Is the OC gain correct?", button name ("OK")="ok") -> (true=w5667:bool)
                            n2448 = local write "OCchecked?"(w5667) -> ()
                          }
                          frame True {
                          }
                        }
                        n2449 = case shown="True" w5666 {
                          frame False {
                          }
                          frame True {
                            n2450 = call "shuttercontrol.vi"("command"="close") -> ()  [unwired: 1 in, 1 out]
                          }
                        }
                        n2451 = call "allAI-temp.vi"("command"=enum16{"get", "set", "clear", "append"}."clear") -> ()  [unwired: 3 in, 2 out]
                      }
                      frame #1 {
                        n2452 = call "sealtestwfparams.vi"("command"="get") -> ("Params out"=w5678:T22)  [unwired: 6 in]
                        n2453 = Unbundle By Name(w5678) -> ("AO parameters"=w5676:T23)
                        n2454 = Index Array(array=w5676, index=0) -> (element=w5675:T24)
                        n2455 = call "generateRampedSquareWave_fromAOparameters.vi"("AO params"=w5675) -> ("Waveform"=w5671:waveform(dbl), "wflength"=w5672:i32)
                        n2456 = Build Array(w5671) -> (w5674:waveform(dbl)[])
                        n2457 = call "waveformssealtestbuffer.vi"("AO wf in"=w5674, "command"="set") -> ()  [unwired: 1 out]
                      }
                      frame #2 {
                        n2458 = local read "Vholding (mV)"() -> (w5681:sgl)
                        n2459 = local read "Current Clamp"() -> (w5687:bool)
                        n2460 = local read "Voltage Clamp"() -> (w5686:bool)
                        n2461 = local read "OCgain"() -> (w5682:sgl)
                        n2462 = local read "CC_ICgain"() -> (w5685:dbl)
                        n2463 = local read "holdon"() -> (w5680:bool)
                        n2464 = call "patchparameters.vi"("command"="get") -> ("Params out"=w5689:T13)  [unwired: 1 in]
                        n2465 = Bundle By Name(cluster=w5689, "VC"=w5686, "CC"=w5687, "CC_icg (pA/mv)"=w5685, "VC_icg (mV/mV)"=10.0, "OCG (mV/pA)"=w5682, "OVG (mV/mV)"=0.1, "Vhold (mV)"=w5681, "holdon"=w5680) -> (w5688:T13)
                        n2466 = call "patchparameters.vi"("Params in"=w5688, "command"="set") -> ()  [unwired: 1 out]
                      }
                    }
                  }
                  frame #1 {
                    w5692 = 2
                    n2467 = call "patchparameters.vi"("command"="get") -> ("Params out"=w5700:T13)  [unwired: 1 in]
                    n2468 = Unbundle By Name(w5700) -> ("holdon"=w5699:bool, "Vhold (mV)"=w5698:sgl, "CC_icg (pA/mv)"=w5706:sgl, "CC"=w5704:bool, "VC_icg (mV/mV)"=w5705:sgl)
                    n2469 = Select(t=w5706, s=w5704, f=w5705) -> (s? t:f=w5707:sgl)
                    n2470 = To Single Precision Float(number=0.001 ("y")) -> (single precision float=w5708:sgl)
                    n2471 = Compound Arithmetic op=MULTIPLY(w5698, w5707, w5708) -> (w5702:sgl)
                    n2472 = case shown="False" w5699 {
                      tunnel: w5702 -> [_ w5720]
                      tunnel: [0.0 w5720] -> w5695
                      frame False {
                      }
                      frame True {
                      }
                    }
                    n2473 = Greater Than 0?(x=w5692) -> (x > 0?=w5694:bool)
                    n2474 = case shown="True" w5694 {
                      tunnel: w5693 -> [_ w5709]
                      tunnel: w5692 -> [_ w5712]
                      frame False {
                      }
                      frame True {
                        n2475 = Initialize Array(sgl 0.0 ("element"), w5712, w5709) -> (w5710:sgl[][])
                        n2476 = call "allAI-temp.vi"("array in"=w5710, "command"=enum16{"get", "set", "clear", "append"}."set") -> ()  [unwired: 2 in, 2 out]
                      }
                    }
                    n2477 = flat-sequence {
                      tunnel: w5693 -> [w5716]
                      tunnel: w5693 -> [w5715]
                      tunnel: [w5715] -> w5697
                      tunnel: [w5714] -> w5696
                      tunnel: w5695 -> [w5714]
                      tunnel: w5697 -> [w5718]
                      tunnel: w5696 -> [w5717]
                      frame #0 {
                        n2478 = call "prepAI_sealtest.vi"("samples per channel"=w5716) -> ()  [unwired: 2 in]
                      }
                      frame #1 {
                        n2479 = call "prepAO_sealtest.vi"("Vhold"=w5717, "samples per channel"=w5718) -> ()  [unwired: 1 in]
                      }
                    }
                  }
                  frame #2 {
                    n2480 = stacked-sequence {
                      frame #0 {
                        n2481 = call "tempconfigAO_seal.vi"("command"="get") -> ("Temp Config out"=w5724:T25)  [unwired: 1 in]
                        n2482 = Unbundle By Name(w5724) -> ("AO"=w5725:refnum<k21>[], "E_AO"=w5726:errorcluster[])
                        n2483 = for {
                          tunnel: w5725 -> [w5734] mode=indexing
                          tunnel: w5726 -> [w5733] mode=indexing
                          tunnel: [w5732] -> w5728 mode=indexing
                          tunnel: [w5731] -> w5729 mode=indexing
                          n2484 = call <vilib>:"DAQmx Start Task.vi"("task/channels in"=w5734, "error in"=w5733) -> ("task out"=w5732:refnum<k21>, "error out"=w5731:errorcluster)  [unwired: 12 in]
                        }
                        n2485 = call "tempconfigAO_seal.vi"("command"="get") -> ("Temp Config out"=w5727:T25)  [unwired: 1 in]
                        n2486 = Bundle By Name(cluster=w5727, "AO"=w5728, "E_AO"=w5729) -> (w5730:T25)
                        n2487 = call "tempconfigAO_seal.vi"("Temp Config in"=w5730, "command"="set") -> ()  [unwired: 1 out]
                      }
                      frame #1 {
                        n2488 = call "tempconfigAI_seal.vi"("command"="get") -> ("Temp Config out"=w5736:T26)  [unwired: 1 in]
                        n2489 = Unbundle By Name(w5736) -> ("AI"=w5741:refnum<k21>, "E_AI"=w5742:errorcluster)
                        n2490 = call <vilib>:"DAQmx Start Task.vi"("task/channels in"=w5741, "error in"=w5742) -> ("task out"=w5743:refnum<k21>, "error out"=w5744:errorcluster)  [unwired: 12 in]
                        n2491 = call "tempconfigAI_seal.vi"("command"="get") -> ("Temp Config out"=w5738:T26)  [unwired: 1 in]
                        n2492 = Bundle By Name(cluster=w5738, "AI"=w5743, "E_AI"=w5744) -> (w5740:T26)
                        n2493 = call "tempconfigAI_seal.vi"("Temp Config in"=w5740, "command"="set") -> ()  [unwired: 1 out]
                      }
                    }
                  }
                  frame #3 {
                    n2494 = while {
                      tunnel: w5745 -> [w5746]
                      stop <- w5747 stop-if-true
                      n2495 = stacked-sequence {
                        seq-local: [_ _ _ w5788 _ _] -> [_ _ _ _ w5840 _]
                        seq-local: [w5749 _ _ _ _ _] -> [_ w5758 _ w5781 w5829 w5860]
                        tunnel: w5746 -> [_ _ w5766 _ w5828 _]
                        frame #0 {
                          n2496 = call "patchparameters.vi"("command"="get") -> ("Params out"=w5756:T13)  [unwired: 1 in]
                          n2497 = local read "Vholding (mV)"() -> (w5753:sgl)
                          n2498 = Unbundle By Name(w5756) -> ("Vhold (mV)"=w5752:sgl, "holdon"=w5755:bool)
                          n2499 = local read "holdon"() -> (w5754:bool)
                          n2500 = Not Equal?(x=w5753, y=w5752) -> (x != y?=w5751:bool)
                          n2501 = Not Equal?(x=w5755, y=w5754) -> (x != y?=w5750:bool)
                          n2502 = Or(x=w5751, y=w5750) -> (x .or. y?=w5749:bool)
                        }
                        frame #1 {
                          n2503 = case shown="True" w5758 {
                            frame False {
                            }
                            frame True {
                              n2504 = local read "Vholding (mV)"() -> (w5761:sgl)
                              n2505 = local read "holdon"() -> (w5759:bool)
                              n2506 = call "patchparameters.vi"("command"="get") -> ("Params out"=w5762:T13)  [unwired: 1 in]
                              n2507 = Bundle By Name(cluster=w5762, "Vhold (mV)"=w5761, "holdon"=w5759) -> (w5760:T13)
                              n2508 = call "patchparameters.vi"("Params in"=w5760, "command"="set") -> ()  [unwired: 1 out]
                            }
                          }
                        }
                        frame #2 {
                          n2509 = call "tempconfigAI_seal.vi"("command"="get") -> ("Temp Config out"=w5776:T26)  [unwired: 1 in]
                          n2510 = Unbundle By Name(w5776) -> ("AI"=w5775:refnum<k21>, "E_AI"=w5774:errorcluster)
                          n2511 = call-poly <vilib>:"DAQmx Read.vi"("task/channels in"=w5775, "number of samples per channel"=w5766, "timeout"=10.0, "error in"=w5774) -> ("task out"=w5770:refnum<k21>, "data"=w5767:i16[][], "error out"=w5779:errorcluster)  [unwired: 9 in]
                          n2512 = call "tempconfigAI_seal.vi"("command"="get") -> ("Temp Config out"=w5771:T26)  [unwired: 1 in]
                          n2513 = Bundle By Name(cluster=w5771, "AI"=w5770, "E_AI"=w5779) -> (w5778:T26)
                          n2514 = To Single Precision Float(number=w5767) -> (single precision float=w5769:sgl[][])
                          n2515 = call "tempconfigAI_seal.vi"("Temp Config in"=w5778, "command"="set") -> ()  [unwired: 1 out]
                          n2516 = call "allAI-temp.vi"("array in"=w5769, "command"=enum16{"get", "set", "clear", "append"}."set") -> ()  [unwired: 2 in, 2 out]
                        }
                        frame #3 {
                          n2517 = case shown="True" w5781 {
                            frame False {
                            }
                            frame True {
                              n2518 = call "tempconfigAO_seal.vi"("command"="get") -> ("Temp Config out"=w5817:T25)  [unwired: 1 in]
                              n2519 = Unbundle By Name(w5817) -> ("AO"=w5816:refnum<k21>[], "E_AO"=w5815:errorcluster[])
                              n2520 = call "tempconfigAI_seal.vi"("command"="get") -> ("Temp Config out"=w5804:T26)  [unwired: 1 in]
                              n2521 = Unbundle By Name(w5804) -> ("AI"=w5805:refnum<k21>, "E_AI"=w5806:errorcluster)
                              n2522 = for {
                                tunnel: w5816 -> [w5821] mode=indexing
                                tunnel: w5815 -> [w5820] mode=indexing
                                tunnel: [w5819] -> w5811 mode=indexing
                                n2523 = call <vilib>:"DAQmx Stop Task.vi"("task/channels in"=w5821, "error in"=w5820) -> ("task out"=w5822:refnum<k21>, "error out"=w5823:errorcluster)  [unwired: 12 in]
                                n2524 = call <vilib>:"DAQmx Clear Task.vi"("task in"=w5822, "error in"=w5823) -> ("error out"=w5819:errorcluster)  [unwired: 13 in]
                              }
                              n2525 = call <vilib>:"DAQmx Stop Task.vi"("task/channels in"=w5805, "error in"=w5806) -> ("task out"=w5802:refnum<k21>, "error out"=w5801:errorcluster)  [unwired: 12 in]
                              n2526 = call <vilib>:"DAQmx Clear Task.vi"("task in"=w5802, "error in"=w5801) -> ("error out"=w5800:errorcluster)  [unwired: 13 in]
                              n2527 = call "tempconfigAO_seal.vi"("command"="get") -> ("Temp Config out"=w5812:T25)  [unwired: 1 in]
                              n2528 = Bundle By Name(cluster=w5812, "E_AO"=w5811) -> (w5810:T25)
                              n2529 = call "tempconfigAI_seal.vi"("command"="get") -> ("Temp Config out"=w5808:T26)  [unwired: 1 in]
                              n2530 = Bundle By Name(cluster=w5808, "E_AI"=w5800) -> (w5799:T26)
                              n2531 = call "tempconfigAO_seal.vi"("Temp Config in"=w5810, "command"="set") -> ()  [unwired: 1 out]
                              n2532 = call "tempconfigAI_seal.vi"("Temp Config in"=w5799, "command"="set") -> ()  [unwired: 1 out]
                            }
                          }
                          n2533 = call "allAI-temp.vi"("command"=enum16{"get", "set", "clear", "append"}."get") -> ("array out"=w5785:sgl[][])  [unwired: 3 in, 1 out]
                          n2534 = call "tempconfigAI_seal.vi"("command"="get") -> ("Temp Config out"=w5797:T26)  [unwired: 1 in]
                          n2535 = Unbundle By Name(w5797) -> ("header"=w5780:dbl[])
                          n2536 = Index Array(array=w5785, index (row) #1=1 ("index (row)"), index (row) #2=0 ("index (row)")) -> (element #1=w5783:sgl[], element #2=w5782:sgl[])  [unwired: 2 in]
                          n2537 = local read "OCgain"() -> (w5790:sgl)
                          n2538 = call "Unscaledtoscaled.vi"("Unscaled Data"=w5783, "Header Information"=w5780) -> ("Array"=w5795:sgl[])  [unwired: 1 in]
                          n2539 = call "Unscaledtoscaled.vi"("Unscaled Data"=w5782, "Header Information"=w5780) -> ("Array"=w5798:sgl[])  [unwired: 1 in]
                          n2540 = Multiply(x=w5795, y=0.1) -> (x*y=w5792:dbl[])
                          n2541 = Divide(x=w5798, y=w5790) -> (x/y=w5791:sgl[])
                          n2542 = Build Array(w5792, w5791) -> (w5794:dbl[][])
                          n2543 = Multiply(x=w5794, y=1000.0) -> (x*y=w5788:dbl[][])
                          "Patch readout" <- w5788
                        }
                        frame #4 {
                          n2544 = case shown="True" w5829 {
                            tunnel: w5828 -> [_ w5841]
                            frame False {
                            }
                            frame True {
                              n2545 = call "patchparameters.vi"("command"="get") -> ("Params out"=w5845:T13)  [unwired: 1 in]
                              n2546 = Unbundle By Name(w5845) -> ("holdon"=w5844:bool, "Vhold (mV)"=w5843:sgl, "CC_icg (pA/mv)"=w5851:sgl, "CC"=w5849:bool, "VC_icg (mV/mV)"=w5850:sgl)
                              n2547 = Select(t=w5851, s=w5849, f=w5850) -> (s? t:f=w5852:sgl)
                              n2548 = To Single Precision Float(number=0.001 ("y")) -> (single precision float=w5853:sgl)
                              n2549 = Compound Arithmetic op=MULTIPLY(w5843, w5852, w5853) -> (w5847:sgl)
                              n2550 = case shown="True" w5844 {
                                tunnel: w5847 -> [_ w5858]
                                tunnel: [0.0 w5858] -> w5842
                                frame False {
                                }
                                frame True {
                                }
                              }
                              n2551 = flat-sequence {
                                tunnel: w5841 -> [w5854]
                                tunnel: w5842 -> [w5856]
                                tunnel: w5841 -> [w5855]
                                frame #0 {
                                n2552 = call "prepAI_sealtest.vi"("samples per channel"=w5854) -> ()  [unwired: 2 in]
                                }
                                frame #1 {
                                n2553 = call "prepAO_sealtest.vi"("Vhold"=w5856, "samples per channel"=w5855) -> ()  [unwired: 1 in]
                                }
                              }
                            }
                          }
                          n2554 = call "sealtestwfparams.vi"("command"="get") -> ("Params out"=w5834:T22)  [unwired: 6 in]
                          n2555 = Unbundle By Name(w5834) -> ("AO parameters"=w5835:T23)
                          n2556 = Index Array(array=w5835, index=0) -> (element=w5837:T24)
                          n2557 = Unbundle By Name(w5837) -> ("Cycles"=w5832:dbl, "Start amplitude (V)"=w5831:dbl, "Sampling frequency (Hz)"=w5830:dbl)
                          n2558 = local read "fitpoints"() -> (w5838:dbl)
                          n2559 = script code="V=data(1,:);\nI=data(2,:);\ntres=mean(V);\nspc=(nsamp./ncyc);\nV=V(spc+1:end-spc);\nI=I(spc+1:end-spc);\ndV=mean(V(V>tres))-mean(V(V<tres))\nIcyc=reshape(I,[spc ncyc-2]);\nIcyc=Icyc';\nIcyc=mean(Icyc,1);\ndIss=mean(Icyc(floor(spc*0.15):floor(spc/2)-2))-mean(Icyc(spc*0.65:spc-2))\nRm=dV*1e3/dIss;\n[maxi,ind]=max(Icyc);\nIfit=Icyc(ind+1:ind+1+points-1)-0.5*(mean(Icyc(floor(spc*0.15):floor(spc/2)-2))+mean(Icyc(spc*0.65:spc-2)))\nt=(3:points-1+3)./srate*1000;\nt=t';\nIfit=Ifit';\nc=fit(t,Ifit, 'exp1');\ncoeffs=coeffvalues(c);\nIa=coeffs(1);\nRa=dV*1e3./Ia/2;\ntau=-1./coeffs(2);\ncap=tau/Ra*1000;"("data"=w5840, "nsamp"=w5828, "ncyc"=w5832, "maxV"=w5831, "points"=w5838, "srate"=w5830) -> ("cap"=w5827:dbl, "Ra"=w5826:dbl, "Icyc"=w5825:dbl[], "Rm"=w5824:dbl)  [unwired: 1 in, 1 out]
                          n2560 = local read "set as Rp?"() -> (w5839:bool)
                          n2561 = local write "Cmembrane"(w5827) -> ()
                          n2562 = local write "Rmembrane (MOhm)"(w5824) -> ()
                          n2563 = local write "Racces (MOhm)"(w5826) -> ()
                          n2564 = case shown="True" w5839 {
                            tunnel: w5824 -> [_ w5859]
                            frame False {
                            }
                            frame True {
                              n2565 = local write "Rpipette (MOhm)"(w5859) -> ()
                            }
                          }
                          n2566 = local write "Ifit"(w5825) -> ()
                        }
                        frame #5 {
                          n2567 = local read "set as Rp?"() -> (w5861:bool)
                          n2568 = case shown="True" w5860 {
                            frame False {
                            }
                            frame True {
                              n2569 = stacked-sequence {
                                frame #0 {
                                n2570 = call "tempconfigAO_seal.vi"("command"="get") -> ("Temp Config out"=w5868:T25)  [unwired: 1 in]
                                n2571 = Unbundle By Name(w5868) -> ("AO"=w5867:refnum<k21>[], "E_AO"=w5866:errorcluster[])
                                n2572 = for {
                                tunnel: w5867 -> [w5875] mode=indexing
                                tunnel: w5866 -> [w5874] mode=indexing
                                tunnel: [w5873] -> w5864 mode=indexing
                                tunnel: [w5872] -> w5863 mode=indexing
                                n2573 = call <vilib>:"DAQmx Start Task.vi"("task/channels in"=w5875, "error in"=w5874) -> ("task out"=w5873:refnum<k21>, "error out"=w5872:errorcluster)  [unwired: 12 in]
                                }
                                n2574 = call "tempconfigAO_seal.vi"("command"="get") -> ("Temp Config out"=w5865:T25)  [unwired: 1 in]
                                n2575 = Bundle By Name(cluster=w5865, "AO"=w5864, "E_AO"=w5863) -> (w5862:T25)
                                n2576 = call "tempconfigAO_seal.vi"("Temp Config in"=w5862, "command"="set") -> ()  [unwired: 1 out]
                                }
                                frame #1 {
                                n2577 = call "tempconfigAI_seal.vi"("command"="get") -> ("Temp Config out"=w5877:T26)  [unwired: 1 in]
                                n2578 = Unbundle By Name(w5877) -> ("AI"=w5882:refnum<k21>, "E_AI"=w5883:errorcluster)
                                n2579 = call <vilib>:"DAQmx Start Task.vi"("task/channels in"=w5882, "error in"=w5883) -> ("task out"=w5884:refnum<k21>, "error out"=w5885:errorcluster)  [unwired: 12 in]
                                n2580 = call "tempconfigAI_seal.vi"("command"="get") -> ("Temp Config out"=w5879:T26)  [unwired: 1 in]
                                n2581 = Bundle By Name(cluster=w5879, "AI"=w5884, "E_AI"=w5885) -> (w5881:T26)
                                n2582 = call "tempconfigAI_seal.vi"("Temp Config in"=w5881, "command"="set") -> ()  [unwired: 1 out]
                                }
                              }
                            }
                          }
                          n2583 = case shown="True" w5861 {
                            frame False {
                            }
                            frame True {
                              n2584 = local write "set as Rp?"(FALSE ("set as Rp?")) -> ()
                            }
                          }
                        }
                      }
                      n2585 = local read "sealtest"() -> (w5748:bool)
                      n2586 = Not(x=w5748) -> (.not. x?=w5747:bool)
                    }
                  }
